vi "DVR.folder.Write.vi"(7 "destination":T1, 8 "error in":errorcluster, 10 "Folder":path, 11 "DVR in":T2) -> (0 "error out":errorcluster)   [LabVIEW 2020]
uses:
  _controls/data.ctl
  camera/camera.lvclass
  _controls/data.ref.ctl
  <vilib>/vision/Image Controls.llb/IMAQ Image.ctl
  _controls/state.ctl
  _controls/data.vars.ctl
  _controls/flip.ctl
  _controls/folder.destination.ctl
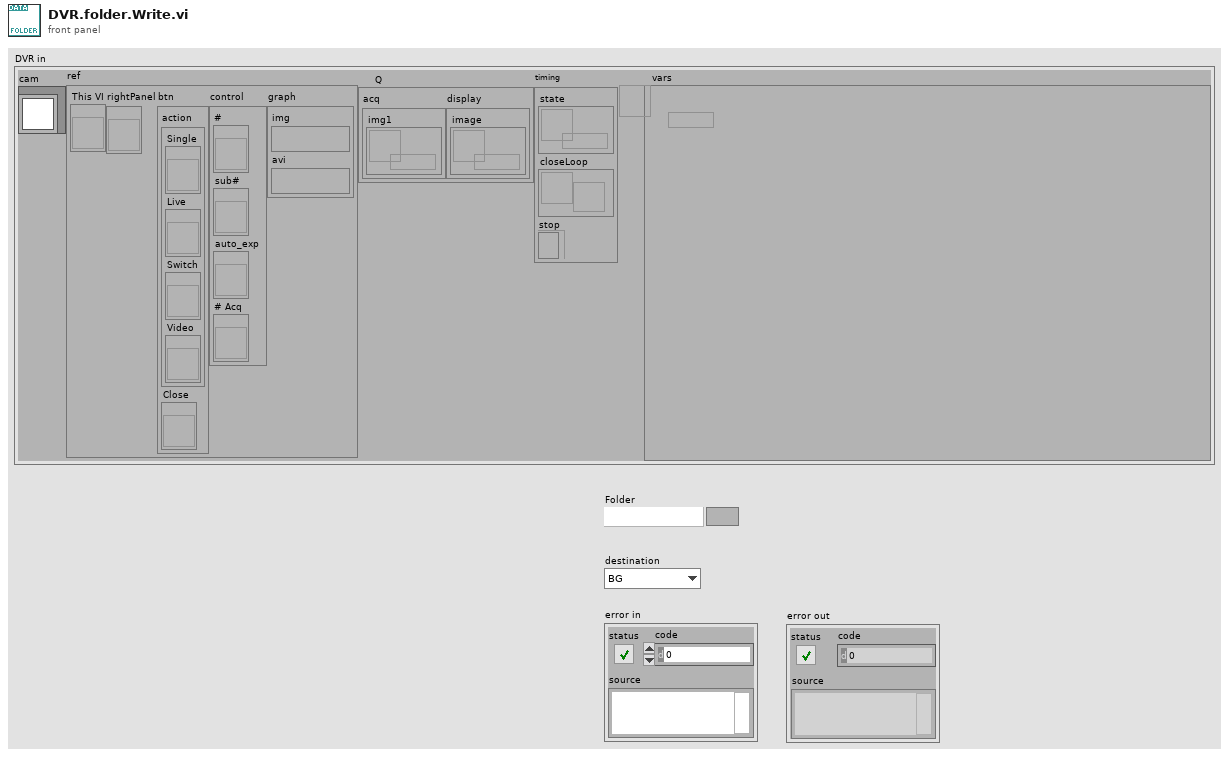
[diagram p1: front panel]
types:
  T1 = typedef "folder.destination.ctl" = enum16{"BG", "FF"}
  T2 = typedef "data.ctl" = cluster{"cam":refnum<class "camera.lvclass">, "ref":T3, "Q":cluster{"acq":cluster{"img1":refnum<queue>}, "display":cluster{"image":refnum<queue>}}, "timing":cluster{"state":refnum<queue>, "closeLoop":refnum<notifier>, "stop":refnum<k4>}, "vars":refnum<data-value>}
  T3 = typedef "data.ref.ctl" = cluster{"This VI":refnum<vi>, "rightPanel":refnum<vi>, "btn":cluster{"action":cluster{"Single":refnum<vi>, "Live":refnum<vi>, "Switch":refnum<vi>, "Video":refnum<vi>}, "Close":refnum<vi>}, "control":cluster{"#":refnum<vi>, "sub#":refnum<vi>, "auto_exp":refnum<vi>, "# Acq":refnum<vi>}, "graph":cluster{"img":T4, "avi":T4}}
  T4 = typedef "IMAQ Image.ctl" = refnum<image>
  T5 = typedef "data.vars.ctl" = cluster{"save":cluster{"base_folder":cluster{"Folder":path, "tif":bool, "jpg":bool}, "module":string, "#":u32, "sub#":u8, "save.op":enum16{"Full", "Light"}, "same?":bool, "Shift":enum16{"Single", "Leapfrog"}, "jpg?":bool, "flip":T6}, "acq":cluster{"# Acq":u16, "rotate":bool, "FPS":dbl}, "calib.manual":cluster{"BG":cluster{"Image":u16[][], "enabled?":bool}, "FF":cluster{"Image":u16[][], "enabled?":bool}}}
  T6 = typedef "flip.ctl" = cluster{"x":bool, "y":bool}
  T7 = typedef "img.u16.graph.25pc.axes.ctl" = u16[][]
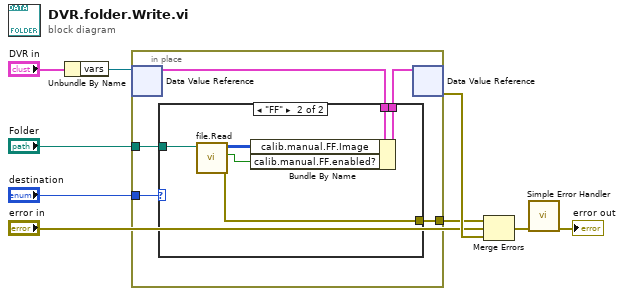
[diagram p0: block diagram]
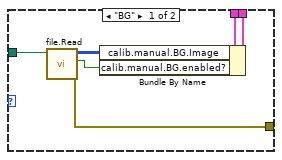
[diagram p2: hidden frame]
diagram:
  n1 = Unbundle By Name("DVR in") -> ("vars"=w8:refnum<data-value>)
  n2 = in-place {
    in-place-border: "destination" -> [w12]
    in-place-border: [w11] -> w3
    in-place-border: "Folder" -> [w10]
    n3 = in-place-dvr #1(w8) -> (w14:T5)  [unwired: 1 out]
    n4 = case shown="\"FF\"" w12 {
      tunnel: w14 -> [w20 w26]
      tunnel: [w19 w25] -> w13
      tunnel: [w15 w22] -> w11
      tunnel: w10 -> [w16 w21]
      frame "BG" {
        n5 = call "file.Read.vi"("Folder"=w16) -> ("error out"=w15:errorcluster, "enabled"=w17:bool, "u16 pixmap"=w18:T7)  [unwired: 8 in]
        n6 = Bundle By Name(cluster=w20, "calib.manual.BG.Image"=w18, "calib.manual.BG.enabled?"=w17) -> (w19:T5)
      }
      frame "FF" {
        n7 = call "file.Read.vi"("Folder"=w21) -> ("error out"=w22:errorcluster, "enabled"=w23:bool, "u16 pixmap"=w24:T7)  [unwired: 8 in]
        n8 = Bundle By Name(cluster=w26, "calib.manual.FF.Image"=w24, "calib.manual.FF.enabled?"=w23) -> (w25:T5)
      }
    }
    n9 = in-place-dvr #1(w13) -> (w9:errorcluster)  [unwired: 1 out]
  }
  n10 = Merge Errors(w3, "error in", w9) -> (w6:errorcluster)
  n11 = call <vilib>:"Simple Error Handler.vi"("error in (no error)"=w6) -> ("error out"=→"error out":errorcluster)  [unwired: 4 in, 4 out]
